vi "Teardown_PanelValueInit.vi"(8 "error in (no error)":errorcluster, 11 "Test.Maui 2.0.Panels in":refnum<class "Test.Maui 2.0.Panels.lvclass">) -> (0 "error out":errorcluster, 3 "Test.Maui 2.0.Panels out":refnum<class "Test.Maui 2.0.Panels.lvclass">)   [LabVIEW 2020, in "Test.Maui 2.0.Panels.lvclass"]
uses:
  Test.Maui 2.0.Panels.lvclass
  Test.Maui 2.0.Panels.lvclass/Test.Maui 2.0.Panels.ctl
  Maui 2.0/Maui 2.0.lvclass
  C:/Program Files (x86)/National Instruments/LabVIEW 2020/vi.lib/JKI/JKI SMO/SMO/SMO.lvclass
  Helper/Test Helper 1/Test Helper 1.lvclass
  <vilib>/JKI/JKI SMO/SMO/SMO.lvclass
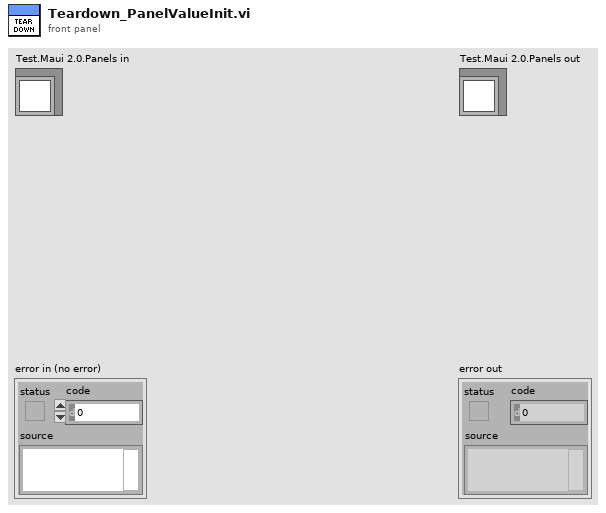
[diagram p1: front panel]
types:
  T1 = cluster{"Stop":refnum<user-event>, "Controls":refnum<user-event>}
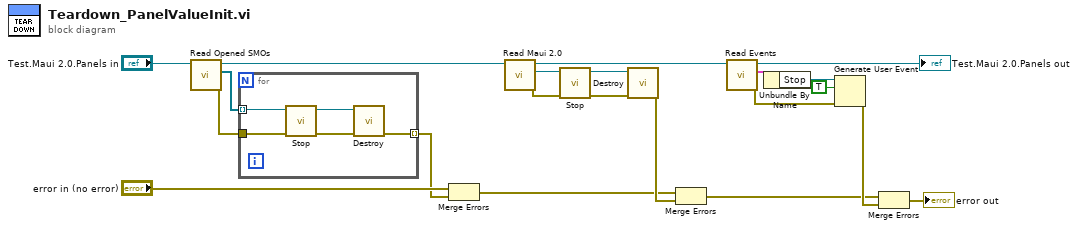
[diagram p0: block diagram]
diagram:
  n1 = call "Read Opened SMOs.vi"("Test.Maui 2.0.Panels in"="Test.Maui 2.0.Panels in") -> ("error out"=w19:errorcluster, "Opened SMOs"=w20:refnum<class "Test Helper 1.lvclass">[], "Test.Maui 2.0.Panels out"=w18:refnum<class "Test.Maui 2.0.Panels.lvclass">)  [unwired: 8 in]
  n2 = for {
    tunnel: w20 -> [w26] mode=indexing
    tunnel: w19 -> [w24]
    tunnel: [w22] -> w7 mode=indexing
    n3 = call <vilib>:"Stop.vi"("error in (no error)"=w24, "SMO"=w26) -> ("error out"=w23:errorcluster, "SMO out"=w25:refnum<class "Test Helper 1.lvclass">)  [unwired: 8 in]
    n4 = call <vilib>:"Destroy.vi"("error in (no error)"=w23, "SMO"=w25) -> ("error out"=w22:errorcluster)  [unwired: 9 in]
  }
  n5 = Merge Errors("error in (no error)", w7) -> (w5:errorcluster)
  n6 = call "Read Maui 2.0.vi"("Test.Maui 2.0.Panels in"=w18) -> ("error out"=w14:errorcluster, "Maui 2.0.lvclass"=w15:refnum<class "Maui 2.0.lvclass">, "Test.Maui 2.0.Panels out"=w13:refnum<class "Test.Maui 2.0.Panels.lvclass">)  [unwired: 8 in]
  n7 = call <vilib>:"Stop.vi"("error in (no error)"=w14, "SMO"=w15) -> ("error out"=w17:errorcluster, "SMO out"=w16:refnum<class "Maui 2.0.lvclass">)  [unwired: 8 in]
  n8 = call <vilib>:"Destroy.vi"("error in (no error)"=w17, "SMO"=w16) -> ("error out"=w6:errorcluster)  [unwired: 9 in]
  n9 = Merge Errors(w5, w6) -> (w3:errorcluster)
  n10 = call "Read Events.vi"("Test.Maui 2.0.Panels in"=w13) -> ("error out"=w2:errorcluster, "Events"=w11:T1, "Test.Maui 2.0.Panels out"=→"Test.Maui 2.0.Panels out":refnum<class "Test.Maui 2.0.Panels.lvclass">)  [unwired: 8 in]
  n11 = Unbundle By Name(w11) -> ("Stop"=w10:refnum<user-event>)
  n12 = Generate User Event(user event=w10, event data cluster=TRUE ("event data"), error in=w2) -> (error out=w4:errorcluster)  [unwired: 1 in, 1 out]
  n13 = Merge Errors(w3, w4) -> (→"error out":errorcluster)
